vi "CreateFolderIfNotExist.vi"(8 "errorIn":errorcluster, 11 "Data Path":path) -> (0 "error out":errorcluster)   [LabVIEW 2011]
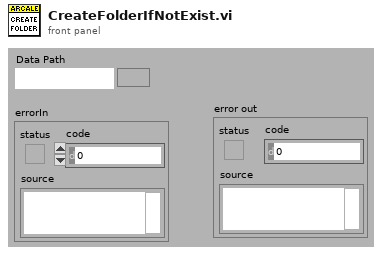
[diagram p1: front panel]
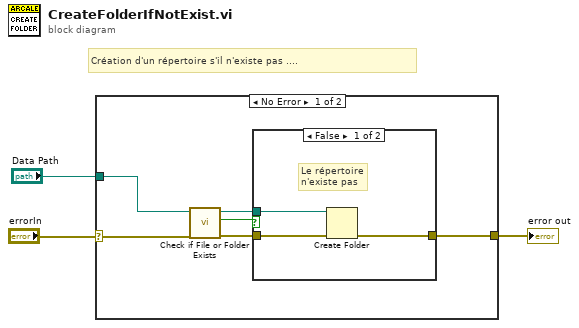
[diagram p0: block diagram]
diagram:
  # "Création d'un répertoire s'il n'existe pas ...."
  n1 = case shown="No Error" "errorIn" {
    selector: "errorIn" -> [w4 w14]
    tunnel: [w9 w14] -> w3
    tunnel: "Data Path" -> [w7 _]
    frame No Error {
      n2 = call <vilib>:"Check if File or Folder Exists.vi"("error in (no error)"=w4, "path"=w7) -> ("error out"=w5:errorcluster, "file or folder exists?"=w8:bool, "dup path"=w6:path)  [unwired: 7 in]
      n3 = case shown="False" w8 {
        tunnel: w5 -> [w12 w13]
        tunnel: w6 -> [w11 _]
        tunnel: [w10 w13] -> w9
        frame False {
          # "Le répertoire\nn'existe pas"
          n4 = Create Folder(path (use dialog)=w11, error in=w12) -> (error out=w10:errorcluster)  [unwired: 1 in, 2 out]
        }
        frame True {
          # "Le répertoire\nexiste !"
        }
      }
    }
    frame Error {
    }
  }
  "error out" <- w3
